vi "sub_SDR_MIMO_AWGN_channel.vi"(7 "Chanel config":T1={"Port 1 -> Port 1"={"Atenuation [dB]"=6.0, "Noise Std. Dev."=0.0, "Initial phase [deg]"=125.0, "Freq. Shift [Hz/Hz]"=0.001}, "Port 1 -> Port 2"={"Atenuation [dB]"=6.0, "Noise Std. Dev."=0.0, "Initial phase [deg]"=125.0, "Freq. Shift [Hz/Hz]"=0.001}, "Port 2 -> Port 1"={"Atenuation [dB]"=6.0, "Noise Std. Dev."=0.0, "Initial phase [deg]"=125.0, "Freq. Shift [Hz/Hz]"=0.001}, "Port 2 -> Port 2"={"Atenuation [dB]"=6.0, "Noise Std. Dev."=0.0, "Initial phase [deg]"=125.0, "Freq. Shift [Hz/Hz]"=0.001}} {"Port 2 -> Port 2"."Freq. Shift [Hz/Hz]" min=0.0 max=1.0 step=0.0001 format="%0.4f"; "Port 2 -> Port 2"."Noise Std. Dev." format="%0.2f"; "Port 2 -> Port 2"."Atenuation [dB]" format="%0.2f"; "Port 2 -> Port 1"."Freq. Shift [Hz/Hz]" min=0.0 max=1.0 step=0.0001 format="%0.4f"; "Port 2 -> Port 1"."Noise Std. Dev." format="%0.2f"; "Port 2 -> Port 1"."Atenuation [dB]" format="%0.2f"; "Port 1 -> Port 2"."Freq. Shift [Hz/Hz]" min=0.0 max=1.0 step=0.0001 format="%0.4f"; "Port 1 -> Port 2"."Noise Std. Dev." format="%0.2f"; "Port 1 -> Port 2"."Atenuation [dB]" format="%0.2f"; "Port 1 -> Port 1"."Freq. Shift [Hz/Hz]" min=0.0 max=1.0 step=0.0001 format="%0.4f"; "Port 1 -> Port 1"."Noise Std. Dev." format="%0.2f"; "Port 1 -> Port 1"."Atenuation [dB]" format="%0.2f"}, 10 "Channel in":cdb[][](array[numeric])) -> (2 "Channel Out":cdb[][](array[numeric]))   [LabVIEW 2012]
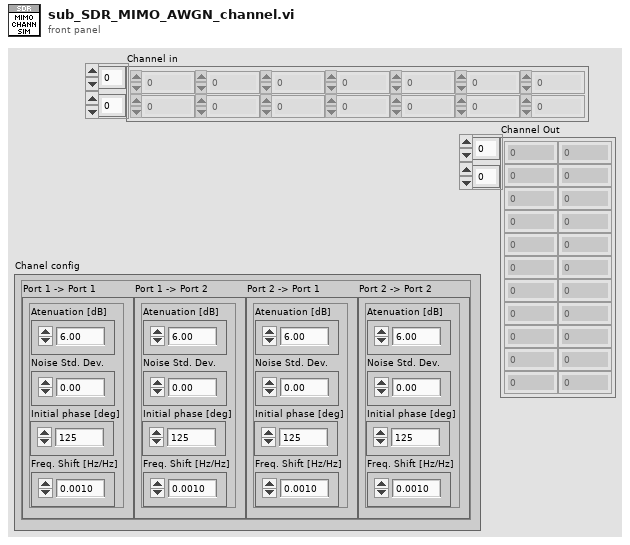
[diagram p1: front panel]
types:
  T1 = cluster{"Port 1 -> Port 1":cluster{"Atenuation [dB]":dbl, "Noise Std. Dev.":dbl, "Initial phase [deg]":dbl, "Freq. Shift [Hz/Hz]":dbl}, "Port 1 -> Port 2":cluster{"Atenuation [dB]":dbl, "Noise Std. Dev.":dbl, "Initial phase [deg]":dbl, "Freq. Shift [Hz/Hz]":dbl}, "Port 2 -> Port 1":cluster{"Atenuation [dB]":dbl, "Noise Std. Dev.":dbl, "Initial phase [deg]":dbl, "Freq. Shift [Hz/Hz]":dbl}, "Port 2 -> Port 2":cluster{"Atenuation [dB]":dbl, "Noise Std. Dev.":dbl, "Initial phase [deg]":dbl, "Freq. Shift [Hz/Hz]":dbl}}
  T2 = cluster{"Atenuation [dB]":dbl, "Noise Std. Dev.":dbl, "Initial phase [deg]":dbl, "Freq. Shift [Hz/Hz]":dbl}
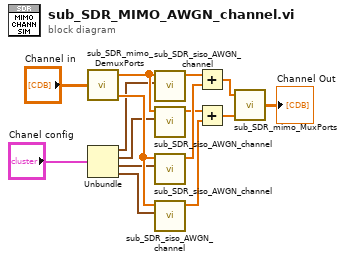
[diagram p0: block diagram]
diagram:
  n1 = call "sub_SDR_mimo_DemuxPorts.vi"("Mux in"="Channel in") -> ("Port 2 out"=w12:cdb[], "Port 1 out"=w13:cdb[])  [unwired: 3 in]
  n2 = Unbundle("Chanel config") -> ("Port 1 -> Port 1"=w4:T2, "Port 1 -> Port 2"=w3:T2, "Port 2 -> Port 1"=w2:T2, "Port 2 -> Port 2"=w1:T2)
  n3 = call "sub_SDR_siso_AWGN_channel.vi"("Channel conf"=w4, "Shaped symbols"=w13) -> ("Array"=w9:cdb[])  [unwired: 9 in]
  n4 = call "sub_SDR_siso_AWGN_channel.vi"("Channel conf"=w3, "Shaped symbols"=w13) -> ("Array"=w7:cdb[])  [unwired: 9 in]
  n5 = call "sub_SDR_siso_AWGN_channel.vi"("Channel conf"=w2, "Shaped symbols"=w12) -> ("Array"=w8:cdb[])  [unwired: 9 in]
  n6 = call "sub_SDR_siso_AWGN_channel.vi"("Channel conf"=w1, "Shaped symbols"=w12) -> ("Array"=w6:cdb[])  [unwired: 9 in]
  n7 = Add(x=w9, y=w8) -> (x+y=w10:cdb[])
  n8 = Add(x=w7, y=w6) -> (x+y=w11:cdb[])
  n9 = call "sub_SDR_mimo_MuxPorts.vi"("Port 2 in"=w11, "Port 1 in"=w10) -> ("Out"=→"Channel Out":cdb[][])  [unwired: 3 in]
